vi "sub_using_token.vi"(8 "error in (no error)":errorcluster, 11 "daq.io type in":T1={"daq.io ref"=refnum, "daq.io API Base"="", "Device Key"="", "Account ID"="", "online"=FALSE, "SSL"=FALSE, "buffer"=TRUE}) -> (0 "error out":errorcluster, 1 "Token ID":string, 2 "using token?":bool, 3 "daq.io type out":T1={"daq.io ref"=refnum, "daq.io API Base"="http://dashboard.daq.io/api/v1", "Device Key"="", "Account ID"="", "online"=TRUE, "SSL"=TRUE, "buffer"=TRUE})   [LabVIEW 2013, in "daqio minimal.lvlib"]
doc: "This VI parses the account ID to determine whether a token is used for authorization and returns the token."
uses:
  daqio minimal.lvlib
  _typedefs/daqio-Type.ctl
  <vilib>/httpClient/ClientHandle.ctl
  <vilib>/httpClient/LabVIEWHTTPClient.lvlib
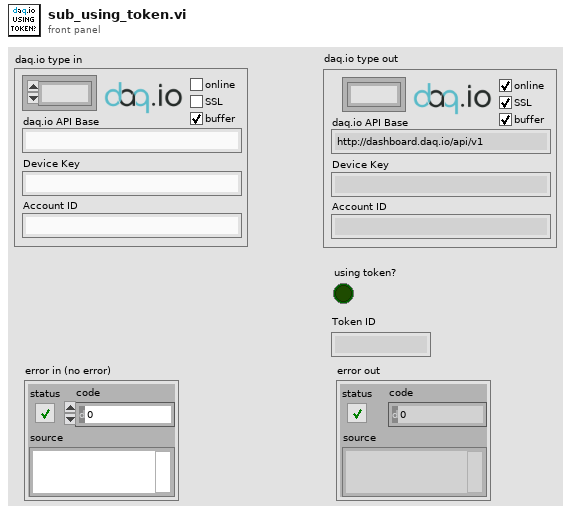
[diagram p1: front panel]
types:
  T1 = typedef "daqio minimal.lvlib/daqio-Type.ctl" = cluster{"daq.io ref":T2, "daq.io API Base":string, "Device Key":string, "Account ID":string, "online":bool, "SSL":bool, "buffer":bool}
  T2 = typedef "LabVIEWHTTPClient.lvlib/ClientHandle.ctl" = refnum<k1>
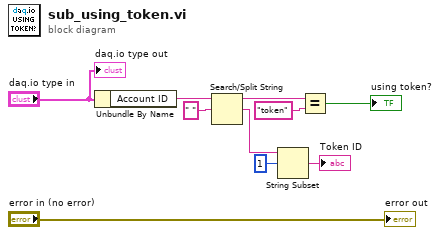
[diagram p0: block diagram]
diagram:
  n1 = Unbundle By Name("daq.io type in") -> ("Account ID"=w9:string)
  n2 = Search/Split String(string=w9, search string/char (-)=" ") -> (substring before match=w10:string, match + rest of string=w3:string)  [unwired: 1 in, 1 out]
  n3 = String Subset(string=w3, offset (0)=1) -> (substring=→"Token ID":string)  [unwired: 1 in]
  n4 = Equal?(x=w10, y="token") -> (x = y?=→"using token?":bool)
  "daq.io type out" <- "daq.io type in"
  "error out" <- "error in (no error)"
